vi "sqrt_calc.vi"() -> ()   [LabVIEW 2020]
panel:
  out "sqrt X":dbl
  in  "X value":dbl
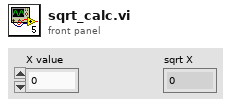
[diagram p1: front panel]
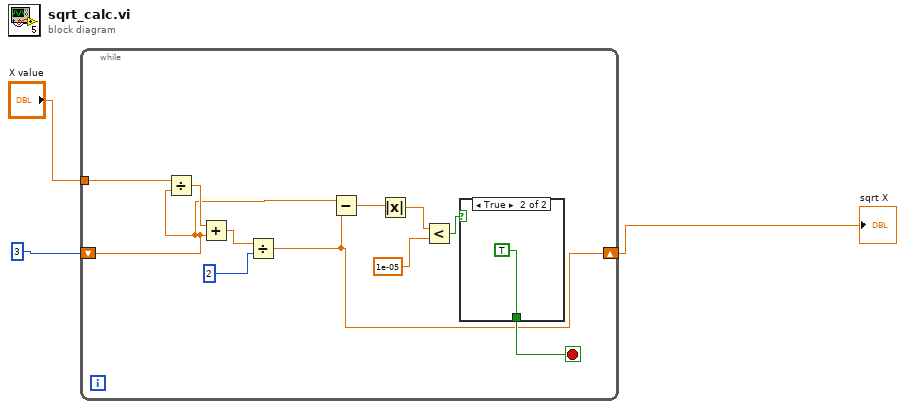
[diagram p0: block diagram]
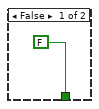
[diagram p2: hidden frame]
diagram:
  n1 = while {
    tunnel: "X value" -> [w14]
    shift-right: [w4] -> w1
    shift-left: 3 -> [w10]
    stop <- w5 stop-if-true
    n2 = Divide(x=w14, y=w10) -> (x/y=w13:dbl)
    n3 = Add(x=w13, y=w10) -> (x+y=w12:dbl)
    n4 = Divide(x=w12, y=2) -> (x/y=w4:dbl)
    n5 = Subtract(x=w10, y=w4) -> (x-y=w9:dbl)
    n6 = Absolute Value(x=w9) -> (abs(x)=w8:dbl)
    n7 = Less?(x=w8, y=1e-05) -> (x < y?=w6:bool)
    n8 = case shown="True" w6 {
      tunnel: [FALSE TRUE] -> w5
      frame False {
      }
      frame True {
      }
    }
  }
  "sqrt X" <- w1
